vi "Serialize - Text.vi"(8 "error in (no error)":errorcluster, 11 "ePAS Data in":refnum<class "ePAS Data.lvclass">) -> (0 "error out":errorcluster, 2 "Serialized Text":string, 3 "ePAS Data out":refnum<class "ePAS Data.lvclass">)   [LabVIEW 2014, in "ePAS Library.lvlib" / "ePAS Data.lvclass"]
uses:
  ePAS Data.lvclass
  ePAS Data.lvclass/ePAS Data.ctl
  reusable/PAS/Data/Main/PAS Data.lvclass
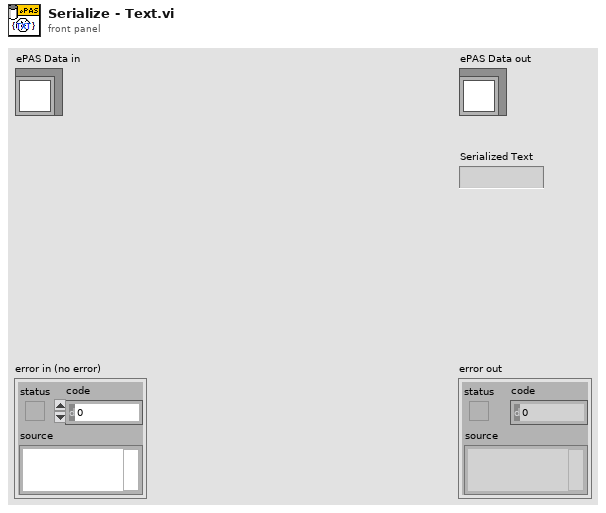
[diagram p1: front panel]
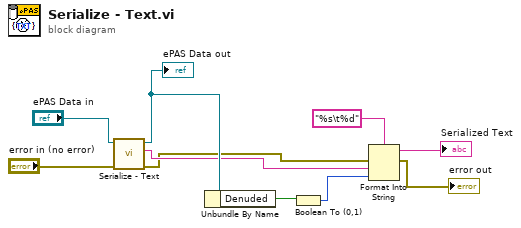
[diagram p0: block diagram]
diagram:
  n1 = call-parent "Serialize - Text.vi"("error in"="error in (no error)", "PAS Data in"="ePAS Data in") -> ("error out"=w2:errorcluster, "Serialized Text"=w5:string, "PAS Data out"=w8:refnum<class "ePAS Data.lvclass">)  [unwired: 7 in]
  "ePAS Data out" <- w8
  n2 = Unbundle By Name(w8) -> ("Denuded"=w7:bool)
  n3 = Boolean To (0,1)(Boolean=w7) -> (0, 1=w4:i16)
  n4 = Format Into String(format string="%s\t%d", error in=w2, w5, w4) -> (resulting string=→"Serialized Text":string, error out=→"error out":errorcluster)  [unwired: 1 in]
